vi "Texture.vi"(4 "Vertical Wrap Mode":enum16{"Clamp", "Repeat"}(ring), 5 "Apply Mode":T2(ring), 6 "Horizontal Wrap Mode":enum16{"Clamp", "Repeat"}(ring), 7 "Filter Mode":T1(ring), 8 "error in (no error)":errorcluster, 10 "path to image":path, 11 "Object in":refnum<class "3D Object.lvclass">) -> (0 "error out":errorcluster, 3 "Object out":refnum<class "3D Object.lvclass">)   [LabVIEW 2015, in "3D Object.lvclass"]
uses:
  3D Object.lvclass
  3D Object.lvclass/3D Object.ctl
  <vilib>/picture/3D Picture Control/NI_3D Picture Control.lvlib
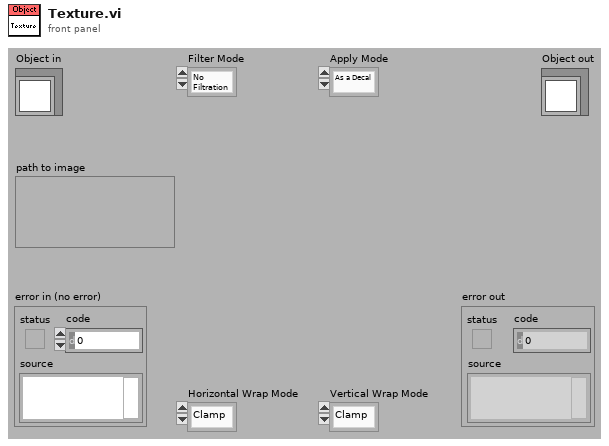
[diagram p1: front panel]
types:
  T1 = enum16{"No Filtration", "Linear Filtration", "Simple Mipmap Filtration", "Bilinear Filtration", "Trilinear Filtration"}
  T2 = enum16{"As a Decal", "With Modulation", "With Blending", "As a replacement"}
  T3 = typedef "imagedata.ctl" = cluster{"image type":i32, "image depth":i32, "image":u8[], "mask":u8[], "colors":u32[], "Rectangle":cluster{"left":i16, "top":i16, "right":i16, "bottom":i16}}
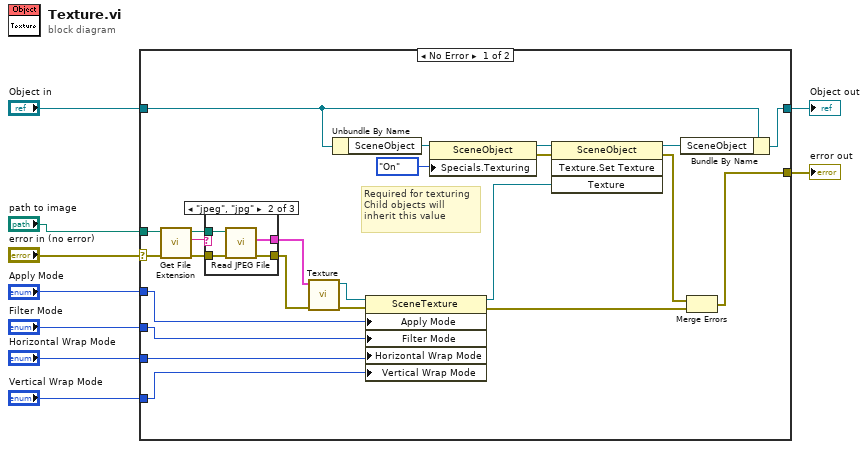
[diagram p0: block diagram]
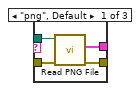
[diagram p2: hidden frame]
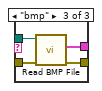
[diagram p3: hidden frame]
diagram:
  n1 = case shown="No Error" "error in (no error)" {
    selector: "error in (no error)" -> [w13 w47]
    tunnel: [w15 w47] -> w9
    tunnel: [w27 w46] -> w7
    tunnel: "Object in" -> [w28 w46]
    tunnel: "Apply Mode" -> [w25 _]
    tunnel: "Filter Mode" -> [w24 _]
    tunnel: "Horizontal Wrap Mode" -> [w23 _]
    tunnel: "Vertical Wrap Mode" -> [w22 _]
    tunnel: "path to image" -> [w14 _]
    frame No Error {
      # "Required for texturing\nChild objects will\ninherit this value"
      n2 = call <vilib>:"Get File Extension.vi"("error in (no error)"=w13, "file"=w14) -> ("error out"=w10:errorcluster, "lowercase file extension"=w12:string, "dup file"=w11:path)  [unwired: 7 out]
      n3 = case shown="\"jpeg\", \"jpg\"" w12 {
        tunnel: [w34 w41 w42] -> w21
        tunnel: [w37 w40 w45] -> w19
        tunnel: w11 -> [w35 w39 w44]
        tunnel: w10 -> [w36 w38 w43]
        frame "png", Default {
          n4 = call <vilib>:"Read PNG File.vi"("error in (no error)"=w36, "path to PNG file"=w35) -> ("error out"=w37:errorcluster, "image data"=w34:T3)  [unwired: 8 out]
        }
        frame "jpeg", "jpg" {
          n5 = call <vilib>:"Read JPEG File.vi"("error in (no error)"=w38, "path to JPEG file"=w39) -> ("error out"=w40:errorcluster, "image data"=w41:T3)  [unwired: 8 out]
        }
        frame "bmp" {
          n6 = call <vilib>:"Read BMP File.vi"("error in (no error)"=w43, "path to BMP file"=w44) -> ("error out"=w45:errorcluster, "image data"=w42:T3)  [unwired: 8 out]
        }
      }
      n7 = call <vilib>:"Texture.vi"("error in (no error)"=w19, "Image"=w21) -> ("error out"=w20:errorcluster, "New Texture Refnum"=w33:refnum<vi>)  [unwired: 8 out]
      n8 = Unbundle By Name(w28) -> ("SceneObject"=w31:refnum<vi>)
      n9 = property class="SceneTexture"(reference=w33, error in=w20, "Apply Mode"=w25, "Filter Mode"=w24, "Horizontal Wrap Mode"=w23, "Vertical Wrap Mode"=w22) -> (reference out=w18:refnum<vi>, error out=w16:errorcluster)
      n10 = property class="SceneObject"(reference=w31, "Specials.Texturing"=enum16{"Inherit Value", "Off", "On"}."On" ("Specials:Texturing")) -> (reference out=w30:refnum<vi>, error out=w29:errorcluster)  [unwired: 1 in]
      n11 = invoke class="SceneObject" method="Texture.Set Texture"(reference=w30, error in=w29, "Texture"=w18) -> (reference out=w26:refnum<vi>, error out=w17:errorcluster)  [unwired: 1 in, 2 out]
      n12 = Bundle By Name(cluster=w28, "SceneObject"=w26) -> (w27:refnum<class "3D Object.lvclass">)
      n13 = Merge Errors(w17, w16) -> (w15:errorcluster)
    }
    frame Error {
    }
  }
  "error out" <- w9
  "Object out" <- w7
